vi "Oscilloscope.vi"() -> ()   [LabVIEW 2015]
panel:
  out "current aquisition":T1
  in  "abort aquisition":bool
  out "Handle Cluster":T2
  out "Progress":string
  out "Actual Length":dbl
  out "Actual Start":dbl
  in  "aquire":bool
  out "current status":T3(ring)
  in  "configure":bool
  in  "Stop Button":bool
  out "error out":errorcluster
  in  "Tab Control":enum32{"channels", "aquisition configuration"}(tab)
  in  "channels \nconfiguration":T4(array[cluster])=[{"Coupling"=0, "Differential Input"=FALSE, "Direct-to-ADC"=FALSE, "Range"=2000, "Impedance"=50, "DC Offset"=0}, {"Coupling"=0, "Differential Input"=FALSE, "Direct-to-ADC"=FALSE, "Range"=2000, "Impedance"=50, "DC Offset"=0}, {"Coupling"=0, "Differential Input"=FALSE, "Direct-to-ADC"=FALSE, "Range"=2000, "Impedance"=50, "DC Offset"=0}, {"Coupling"=0, "Differential Input"=FALSE, "Direct-to-ADC"=FALSE, "Range"=2000, "Impedance"=50, "DC Offset"=0}] {"Impedance" min=50 max=1000000 step=999950; "Coupling" items=["DC", "AC"]}
  in  "Continuous":bool
  in  "Trigger":T5={"Slope"=0, "Level"=0, "Source"=0, "External Range"=2000, "External Coupling"=0, "External"=FALSE, "Disable"=FALSE, "External Impedance"=1} {"External Impedance" items=["50 Ohm", "HiZ"]; "External Coupling" items=["DC", "AC"]; "External Range" min=2000 max=10000 step=8000; "Slope" items=["Rising", "Falling"]; "Level" min=-100 max=100; "Source" min=0 max=64 step=1}
  in  "Acquisition":T1={"Sample Rate"=1000000.0, "Clock mode"=enum."Internal", "Mode"=0, "post trigger"=8192.0, "Segment Size"=8192.0, "Trigger Timeout"=100000.0, "Trigger Holdoff"=0.0, "Trigger Delay"=0.0, "number of records"=0} {"Segment Size" min=256.0 step=128.0; "Trigger Holdoff" min=0.0 step=128.0; "Trigger Delay" min=0.0 step=128.0; "post trigger" min=256.0 step=128.0; "Mode" items=["Single", "Dual", "Quad", "Octal"]}
  out "System:":string
  out "system information":T6
  out "Waveform Graph":T7(graph)
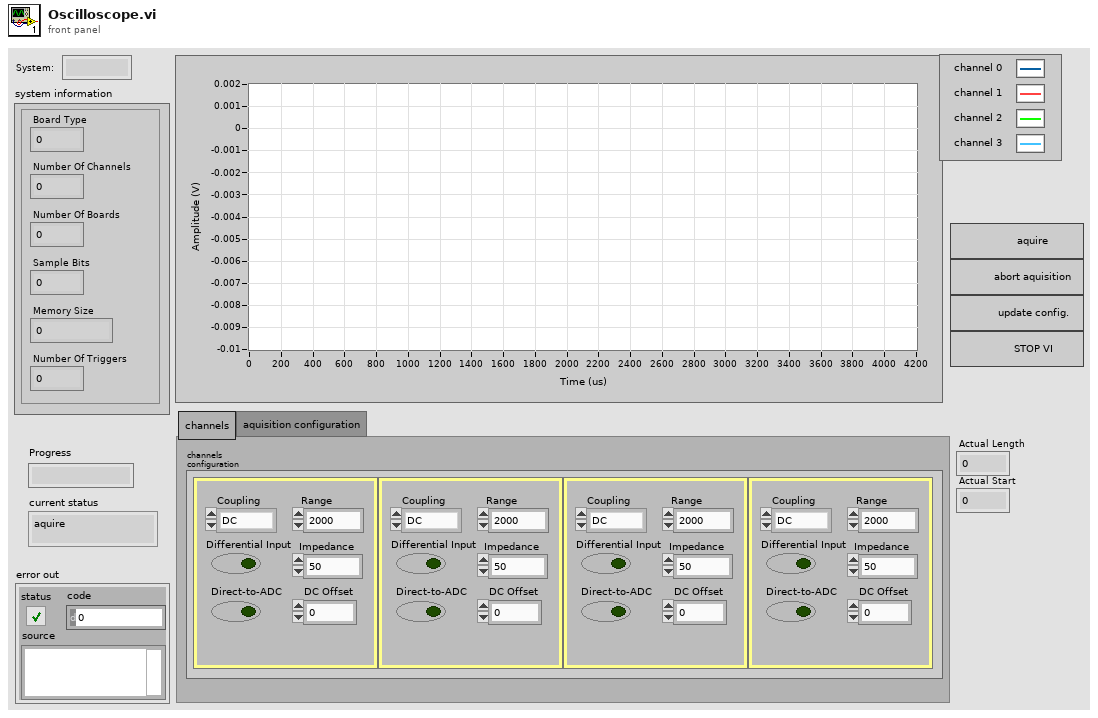
[diagram p1: front panel]
types:
  T1 = cluster{"Sample Rate":dbl, "Clock mode":enum16{"Internal", "External", "Reference"}, "Mode":u16, "post trigger":dbl, "Segment Size":dbl, "Trigger Timeout":dbl, "Trigger Holdoff":dbl, "Trigger Delay":dbl, "number of records":u32}
  T2 = cluster{"Handle":u32, "Sample size":u32, "Resolution":i32, "Offset":i32, "Channels":u32, "Boards":u32}
  T3 = enum16{"aquire", "configure acquisition", "stop VI", "wait"}
  T4 = cluster{"Coupling":u16, "Differential Input":bool, "Direct-to-ADC":bool, "Range":u32, "Impedance":u32, "DC Offset":i32}[]
  T5 = cluster{"Slope":u16, "Level":i32, "Source":i32, "External Range":u32, "External Coupling":u16, "External":bool, "Disable":bool, "External Impedance":u16}
  T6 = cluster{"Memory Size":dbl, "Board Type":u32, "Number Of Channels":u32, "Number Of Boards":u32, "Sample Bits":u32, "Number Of Triggers":u32}
  T7 = cluster{"Actual Start":dbl, dbl, "Data in Volts":dbl[][]}
  T8 = enum8{"Enabled", "Disabled", "Disabled and Grayed Out"}
  T9 = enum16{"aquire", "configure acquisition", "stop VI", "wait"}[]
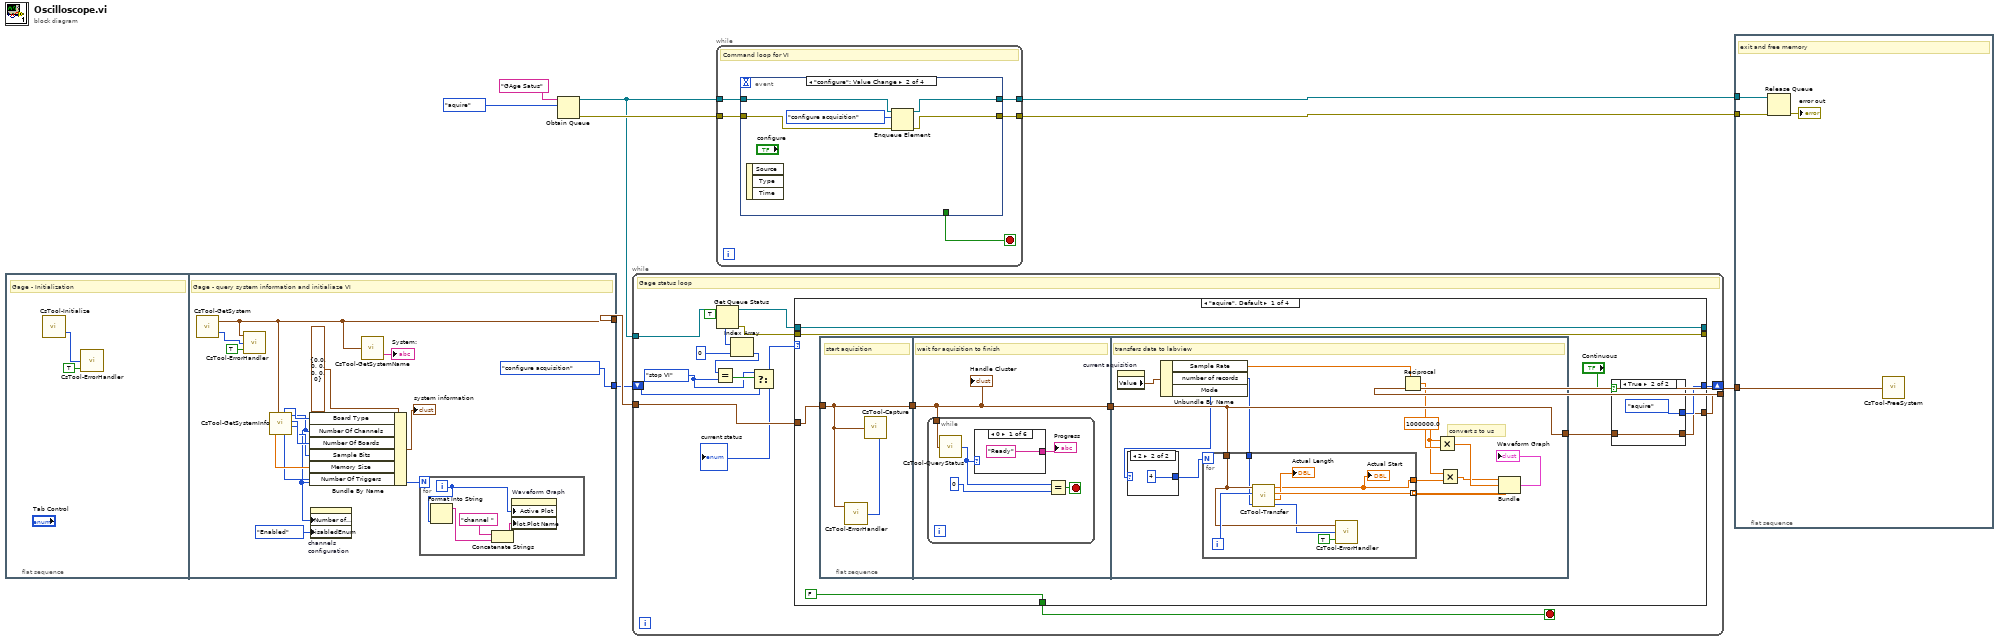
[diagram p0: block diagram]
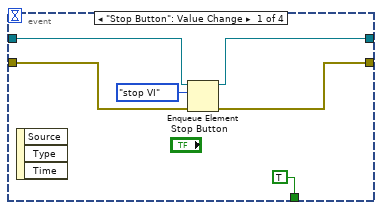
[diagram p2: hidden frame]
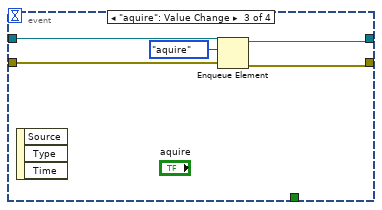
[diagram p3: hidden frame]
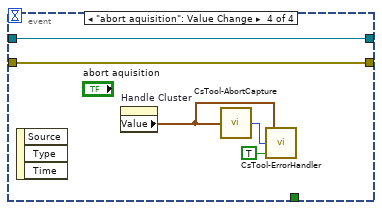
[diagram p4: hidden frame]
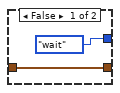
[diagram p5: hidden frame]
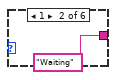
[diagram p6: hidden frame]
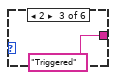
[diagram p7: hidden frame]
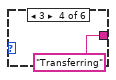
[diagram p8: hidden frame]
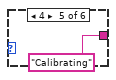
[diagram p9: hidden frame]
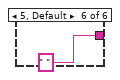
[diagram p10: hidden frame]
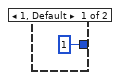
[diagram p11: hidden frame]
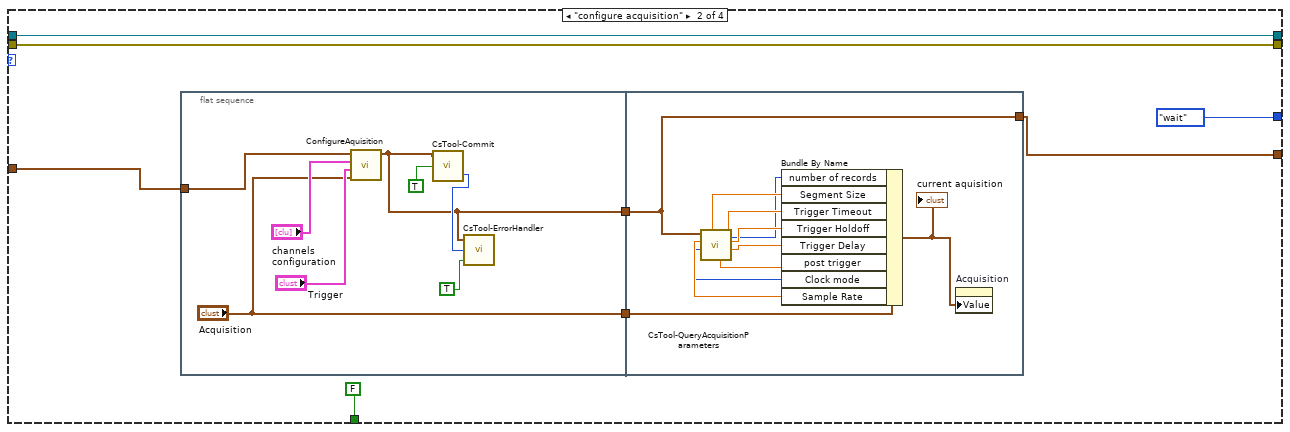
[diagram p12: hidden frame]
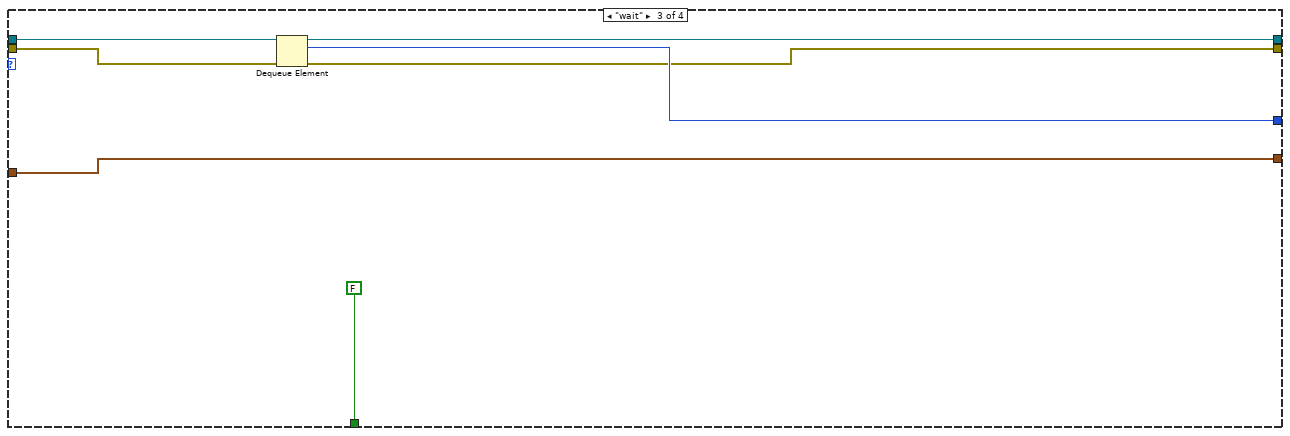
[diagram p13: hidden frame]
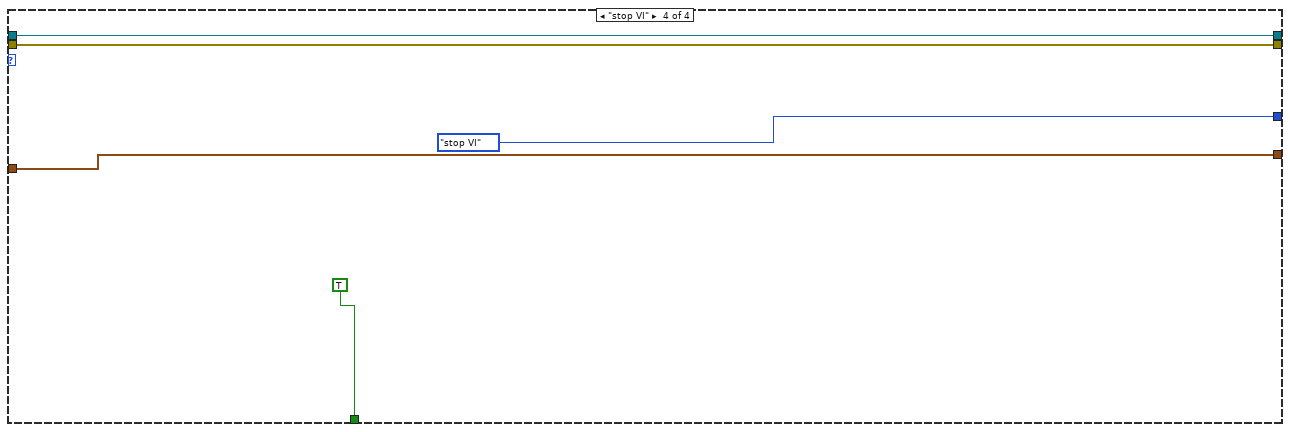
[diagram p14: hidden frame]
diagram:
  n1 = flat-sequence {
    tunnel: [w15] -> w9
    tunnel: [T3."configure acquisition"] -> w1
    frame #0 {
      # "Gage - Initialization"
      n2 = call <userlib>:"CsTool-Initialize.vi"() -> ("Error Code"=w11:i32)  [unwired: 1 out]
      n3 = call <userlib>:"CsTool-ErrorHandler.vi"("StopOnError (true)"=TRUE, "Error Code"=w11) -> ()  [unwired: 1 in, 1 out]
    }
    frame #1 {
      # "Gage - query system information and initialiaze VI"
      n4 = call <userlib>:"CsTool-GetSystem.vi"() -> ("Error Code"=w13:i32, "Handle Cluster"=w15:T2)  [unwired: 4 in]
      n5 = call <userlib>:"CsTool-ErrorHandler.vi"("StopOnError (true)"=TRUE, "Error Code"=w13, "Handle Cluster"=w15) -> ()  [unwired: 1 out]
      n6 = call <userlib>:"CsTool-GetSystemInfo.vi"("Handle Cluster"=w15) -> ("Memory Size"=w22:dbl, "Board Type"=w25:u32, "Number Of Triggers"=w20:u32, "Number Of Channels"=w16:u32, "Number Of Boards"=w24:u32, "Sample Bits"=w23:u32)  [unwired: 1 out]
      n7 = Bundle By Name(cluster=T6 {"Memory Size"=0.0, "Board Type"=0, "Number Of Channels"=0, "Number Of Boards"=0, "Sample Bits"=0, "Number Of Triggers"=0} ("system information"), "Board Type"=w25, "Number Of Channels"=w16, "Number Of Boards"=w24, "Sample Bits"=w23, "Memory Size"=w22, "Number Of Triggers"=w20) -> (→"system information":T6)
      n8 = property on="channels \nconfiguration" class="Arr (strict)"("Number of Columns"=w16, "DisabledEnum"=T8."Enabled" ("Disabled")) -> ()  [unwired: 2 in, 2 out]
      n9 = call <userlib>:"CsTool-GetSystemName.vi"("Handle Cluster"=w15) -> ("System Name"=→"System:":string)  [unwired: 1 out]
      n10 = for {
        N: w16 -> [_]
        i -> [w28]
        n11 = Format Into String(w28) -> (resulting string=w27:string)  [unwired: 3 in, 1 out]
        n12 = Concatenate Strings("channel ", w27) -> (w26:string)
        n13 = property on="Waveform Graph" class="WFGraph (strict)"("Active Plot"=w28, "Plot.Plot Name"=w26) -> ()  [unwired: 2 in, 2 out]
      }
    }
  }
  n14 = Obtain Queue(name (unnamed)="GAge Satus", element data type=T3."aquire") -> (queue out=w2:refnum<queue>, error out=w6:errorcluster)  [unwired: 3 in, 1 out]
  n15 = while {
    tunnel: w9 -> [w39]
    tunnel: [w38] -> w8
    tunnel: w2 -> [w44]
    shift-right: [w31] -> _
    shift-left: w1 -> [w37]
    stop <- w42 stop-if-true
    w33 = T3."stop VI"
    # "Gage status loop"
    n16 = Get Queue Status(queue=w44, return elements? (F)=TRUE) -> (queue out=w40:refnum<queue>, error out=w30:errorcluster, elements=w43:T9)  [unwired: 1 in, 5 out]
    n17 = Index Array(array=w43, index=0) -> (element=w34:T3)
    n18 = Equal?(x=w34, y=w33) -> (x = y?=w35:bool)
    n19 = Select(t=w33, s=w35, f=w37) -> (s? t:f=w32:T3)
    "current status" <- w32
    n20 = case shown="\"aquire\", Default" w32 {
      tunnel: [FALSE FALSE FALSE TRUE] -> w42
      tunnel: [w53 w102 w127 w133] -> _
      tunnel: w40 -> [w53 w102 w128 w133]
      tunnel: w39 -> [w51 w101 w129 w132]
      tunnel: [w46 w97 w129 w132] -> w38
      tunnel: [w48 T3."wait" w126 T3."stop VI"] -> w31
      tunnel: w30 -> [w52 w99 w125 w130]
      tunnel: [w52 w99 w124 w130] -> _
      frame "aquire", Default {
        n21 = flat-sequence {
          tunnel: w51 -> [w59]
          tunnel: [w59] -> w50
          tunnel: w50 -> [w61]
          tunnel: [w61] -> w49
          tunnel: w49 -> [w85]
          tunnel: [w85] -> w47
          frame #0 {
            # "start aquisition"
            n22 = call <userlib>:"CsTool-Capture.vi"("Handle Cluster"=w59) -> ("Error Code"=w60:i32)
            n23 = call <userlib>:"CsTool-ErrorHandler.vi"("Error Code"=w60, "Handle Cluster"=w59) -> ()  [unwired: 1 in, 1 out]
          }
          frame #1 {
            # "wait for aquisition to finish"
            n24 = while {
              tunnel: w61 -> [w63]
              stop <- w62 stop-if-true
              n25 = call <userlib>:"CsTool-QueryStatus.vi"("Handle Cluster"=w63) -> ("Status"=w65:i32)
              n26 = case shown="0" w65 {
                tunnel: ["Ready" "Waiting" "Triggered" "Transferring" "Calibrating" " "] -> w66
                frame 0 {
                }
                frame 1 {
                }
                frame 2 {
                }
                frame 3 {
                }
                frame 4 {
                }
                frame 5, Default {
                }
              }
              "Progress" <- w66
              n27 = Equal?(x=w65, y=0) -> (x = y?=w62:bool)
            }
            "Handle Cluster" <- w61
          }
          frame #2 {
            w78 = 1000000.0 ("x")
            # "convert s to us"
            # "transfers data to labview"
            n28 = property on="current aquisition" class="Clust (strict)"() -> ("Value"=w74:T1)  [unwired: 2 in, 2 out]
            n29 = Unbundle By Name(w74) -> ("Sample Rate"=w83:dbl, "number of records"=w75:u32, "Mode"=w73:u16)
            n30 = case shown="2" w73 {
              tunnel: [1 4] -> w76
              frame 1, Default {
              }
              frame 2 {
              }
            }
            n31 = for {
              N: w76 -> [_]
              tunnel: w85 -> [w92]
              tunnel: [w94] -> w77 mode=indexing
              tunnel: [w89] -> w80
              tunnel: w75 -> [w88]
              i -> [w95]
              n32 = call <userlib>:"CsTool-Transfer.vi"("Segment (1)"=w88, "Channel (0)"=w95, "Handle Cluster"=w92) -> ("Error Code"=w91:i32, "Actual Length"=→"Actual Length":dbl, "Data in Volts"=w94:dbl[], "Actual Start"=w89:dbl)  [unwired: 3 in]
              "Actual Start" <- w89
              n33 = call <userlib>:"CsTool-ErrorHandler.vi"("StopOnError (true)"=TRUE, "Error Code"=w91, "Handle Cluster"=w92) -> ()  [unwired: 1 out]
            }
            n34 = Reciprocal(x=w83) -> (1/x=w82:dbl)
            n35 = Multiply(x=w78, y=w82) -> (x*y=w81:dbl)
            n36 = Multiply(x=w78, y=w80) -> (x*y=w79:dbl)
            n37 = Bundle(w79, w81, "Data in Volts"=w77) -> (→"Waveform Graph":cluster{dbl, dbl, "Data in Volts":dbl[][]})  [unwired: 1 in]
          }
        }
        n38 = case shown="True" "Continuous" {
          tunnel: [T3."wait" T3."aquire"] -> w48
          tunnel: w47 -> [w55 w57]
          tunnel: [w55 w57] -> w46
          frame False {
          }
          frame True {
          }
        }
      }
      frame "configure acquisition" {
        n39 = flat-sequence {
          tunnel: w101 -> [w111]
          tunnel: [w106] -> w98
          tunnel: ["Acquisition"] -> w96
          tunnel: [w122] -> w97
          tunnel: w98 -> [w122]
          tunnel: w96 -> [w121]
          frame #0 {
            n40 = call "ConfigureAquisition.vi"("Acquisition"="Acquisition", "Trigger"="Trigger", "channels configuration"="channels \nconfiguration", "Handle Cluster"=w111) -> ("Handle Cluster 2"=w106:T2)  [unwired: 6 in, 1 out]
            n41 = call <userlib>:"CsTool-Commit.vi"("Coerce Flag (f)"=TRUE, "Handle Cluster"=w106) -> ("Error Code"=w107:i32)  [unwired: 1 in, 1 out]
            n42 = call <userlib>:"CsTool-ErrorHandler.vi"("StopOnError (true)"=TRUE, "Error Code"=w107, "Handle Cluster"=w106) -> ()  [unwired: 1 out]
          }
          frame #1 {
            n43 = call <userlib>:"CsTool-QueryAcquisitionParameters.vi"("Handle Cluster"=w122) -> ("Trigger Delay"=w117:dbl, "Trigger Holdoff"=w116:dbl, "Trigger Timeout"=w115:dbl, "Depth"=w118:dbl, "Segment Count"=w112:u32, "Segment Size"=w114:dbl, "Clock Mode"=w119:enum16{"Internal", "External", "Reference"}, "Sample Rate"=w120:dbl)  [unwired: 3 out]
            n44 = Bundle By Name(cluster=w121, "number of records"=w112, "Segment Size"=w114, "Trigger Timeout"=w115, "Trigger Holdoff"=w116, "Trigger Delay"=w117, "post trigger"=w118, "Clock mode"=w119, "Sample Rate"=w120) -> (w113:T1)
            "current aquisition" <- w113
            n45 = property on="Acquisition" class="Clust (strict)"("Value"=w113) -> ()  [unwired: 2 in, 2 out]
          }
        }
      }
      frame "wait" {
        n46 = Dequeue Element(queue=w128, error in (no error)=w125) -> (queue out=w127:refnum<queue>, element=w126:T3, error out=w124:errorcluster)  [unwired: 1 in, 1 out]
      }
      frame "stop VI" {
      }
    }
  }
  n47 = while {
    tunnel: w6 -> [w138]
    tunnel: w2 -> [w139]
    tunnel: [w137] -> w4
    tunnel: [w136] -> w3
    stop <- w135 stop-if-true
    # "Command loop for VI"
    n48 = event shown="[1] \"configure\": Value Change" {
      selector: _ -> [_ _ _ _]
      dyn-events: _ -> [_ _ _ _]
      timeout: _ -> [_ _ _ _]
      tunnel: w139 -> [w145 w150 w155 w159]
      tunnel: w138 -> [w144 w147 w153 w160]
      tunnel: [w142 w149 w154 w159] -> w137
      tunnel: [w141 w148 w152 w160] -> w136
      tunnel: [TRUE _ _ _] -> w135
      event "Stop Button": Value Change {
        n49 = event-data() -> ()  [unwired: 1 in, 3 out]
        n50 = Enqueue Element(queue=w145, element=T3."stop VI", error in (no error)=w144) -> (queue out=w142:refnum<queue>, error out=w141:errorcluster)  [unwired: 1 in, 1 out]
      }
      event "configure": Value Change {
        n51 = event-data() -> ()  [unwired: 1 in, 3 out]
        n52 = Enqueue Element(queue=w150, element=T3."configure acquisition", error in (no error)=w147) -> (queue out=w149:refnum<queue>, error out=w148:errorcluster)  [unwired: 1 in, 1 out]
      }
      event "aquire": Value Change {
        n53 = event-data() -> ()  [unwired: 1 in, 3 out]
        n54 = Enqueue Element(queue=w155, element=T3."aquire", error in (no error)=w153) -> (queue out=w154:refnum<queue>, error out=w152:errorcluster)  [unwired: 1 in, 1 out]
      }
      event "abort aquisition": Value Change {
        n55 = event-data() -> ()  [unwired: 1 in, 3 out]
        n56 = property on="Handle Cluster" class="Clust (strict)"() -> ("Value"=w157:T2)  [unwired: 2 in, 2 out]
        n57 = call <userlib>:"CsTool-AbortCapture.vi"("Handle Cluster"=w157) -> ("Error Code"=w158:i32)
        n58 = call <userlib>:"CsTool-ErrorHandler.vi"("StopOnError (true)"=TRUE, "Error Code"=w158, "Handle Cluster"=w157) -> ()  [unwired: 1 out]
      }
    }
  }
  n59 = flat-sequence {
    tunnel: w8 -> [w164]
    tunnel: w4 -> [w163]
    tunnel: w3 -> [w162]
    frame #0 {
      # "exit and free memory"
      n60 = Release Queue(queue=w163, error in (no error)=w162) -> (error out=→"error out":errorcluster)  [unwired: 1 in, 2 out]
      n61 = call <userlib>:"CsTool-FreeSystem.vi"("Handle Cluster"=w164) -> ()  [unwired: 1 out]
    }
  }
